vi "AcquireBurstModeData.vi"(7 "Watchdog":refnum<data-value>, 8 "error in (no error)":errorcluster, 11 "config in":T5 {"HighPassFilterState"."Filter State" format="%.2f"; "HighPassFilterState"."IIR Filter Cluster"."Forward Coefficients" format="%.2f"; "HighPassFilterState"."IIR Filter Cluster"."Reverse Coefficients" format="%.2f"; "FixedSizeX32"."InputConfig" items=["AC Coupled", "DC Coupled", "IEPE AC Coupled"]}) -> (0 "error out":errorcluster, 1 "burst mode dataflow messages":T1[](array[typedef]), 3 "config out":T5 {"HighPassFilterState"."Filter State" format="%.2f"; "HighPassFilterState"."IIR Filter Cluster"."Forward Coefficients" format="%.2f"; "HighPassFilterState"."IIR Filter Cluster"."Reverse Coefficients" format="%.2f"; "FixedSizeX32"."InputConfig" items=["AC Coupled", "DC Coupled", "IEPE AC Coupled"]})   [LabVIEW 2017, in "CmsAcquisition.lvlib"]
uses:
  <vilib>/addons/InsightCM/Devices/Shared/Cms/CmsAcquisition/CmsAcquisition.lvlib
  <vilib>/addons/InsightCM/Devices/Shared/Cms/CmsAcquisition/controls/Configuration.ctl
  <vilib>/addons/InsightCM/Devices/Shared/Cms/CmsAcquisition/controls/TachometerConfig.ctl
  <vilib>/addons/InsightCM/Devices/Shared/Cms/CmsAcquisition/controls/FixedSizeArrays.ctl
  <vilib>/LabVIEW Targets/FPGA/cRIO/shared/nicrio_ModuleControls/nicrio_cRIO-9232_ConfigModeRing.ctl
  <vilib>/addons/InsightCM/Devices/Shared/Cms/cRIOWfmAcq/subVIs/RIO Wfm Cust Ctrls/rwfm_SamplingInfo.ctl
  <vilib>/addons/InsightCM/Devices/Shared/Cms/CmsAcquisition/controls/Group.ctl
  <vilib>/addons/InsightCM/Devices/Shared/Cms/CmsAcquisition/controls/Channel.ctl
  <vilib>/addons/InsightCM/Utilities/Analysis/Vibration/controls/HighPassFilterState.ctl
  <vilib>/addons/InsightCM/Devices/Shared/Cms/CmsAcquisition/controls/BurstMode.ctl
  <vilib>/addons/InsightCM/Devices/Shared/Common/DataFlow/controls/Data.ctl
  <vilib>/addons/InsightCM/Utilities/DataAccessors/controls/wfmSGL_DVR.ctl
  <vilib>/addons/PointValueMap/controls/PointMap.ctl
  <vilib>/addons/InsightCM/Devices/Shared/Common/DataFlow/controls/Type.ctl
  <vilib>/NI/Software Watchdog/Watchdog/Watchdog.lvclass
  <vilib>/addons/InsightCM/Utilities/Analysis/Shared/controls/PulsePositions.ctl
  <vilib>/addons/InsightCM/Utilities/Analysis/Shared/AnalysisHelper.lvlib
  <vilib>/addons/PointValueMap/PointValueMap.lvlib
  <vilib>/addons/InsightCM/Devices/Shared/Common/DataFlow/DataFlow.lvlib
  <vilib>/addons/InsightCM/Devices/Shared/Cms/cRIOWfmAcq/cRIOWfmLib.lvlib
  <vilib>/addons/InsightCM/Utilities/Analysis/Vibration/VibrationAnalysisFunctions.lvlib
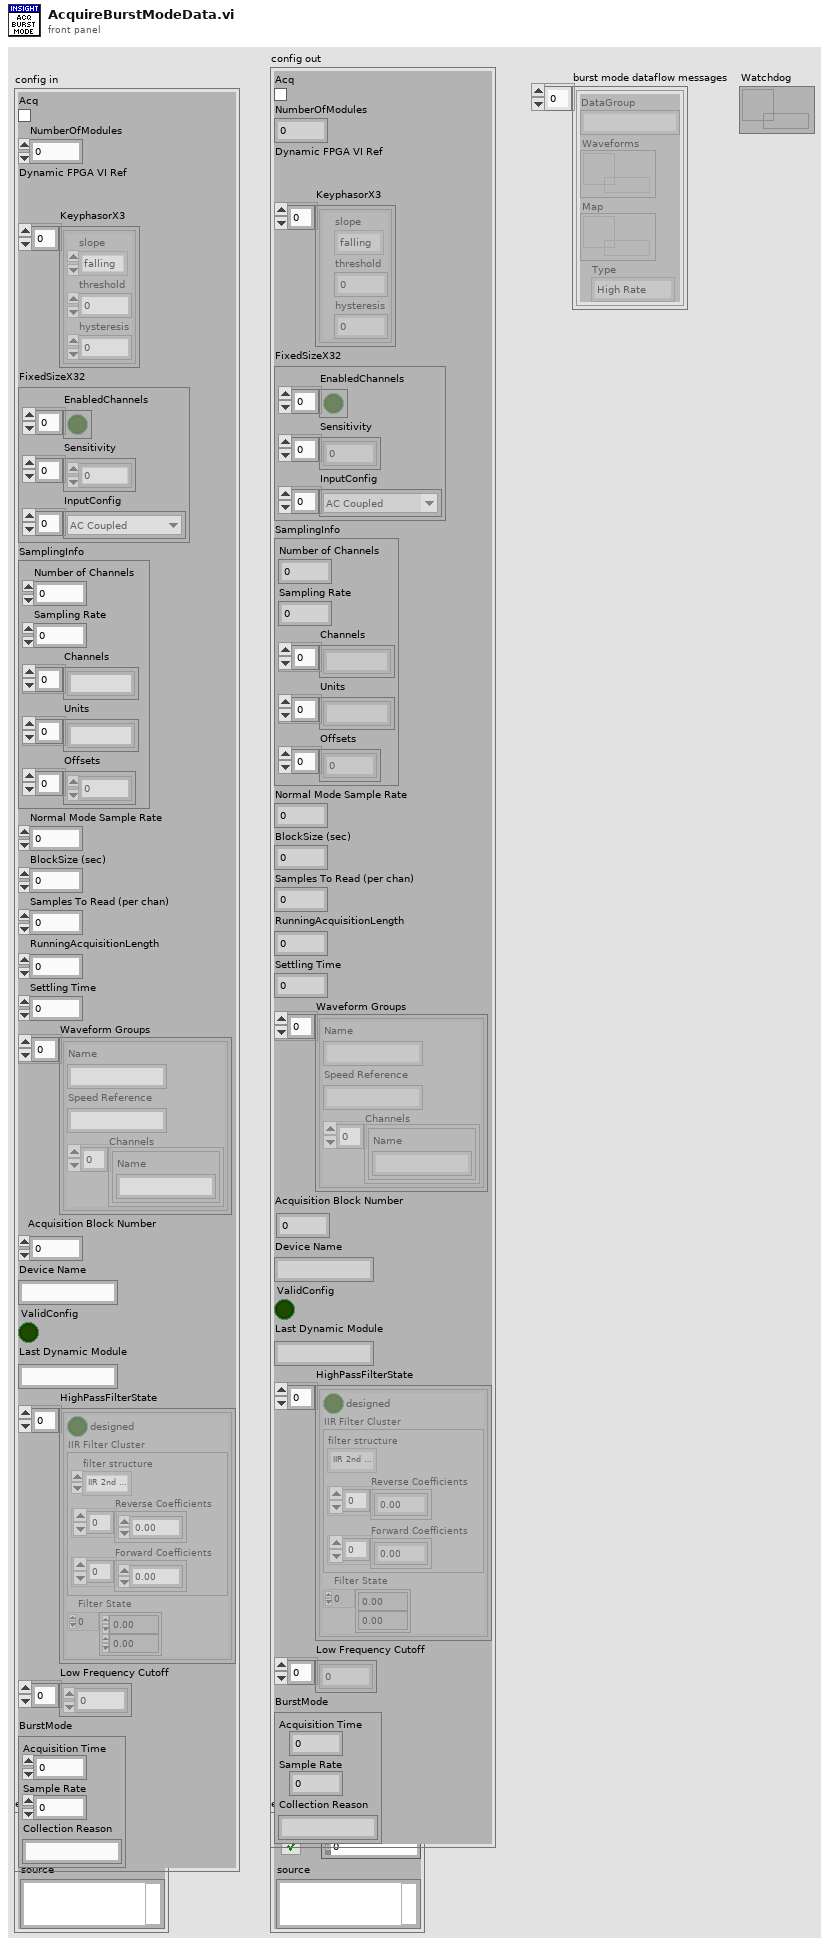
[diagram p1: front panel]
types:
  T1 = typedef "DataFlow.lvlib/Data.ctl" = cluster{"DataGroup":string, "Waveforms":T2, "Map":T3, "Type":T4}
  T2 = typedef "wfmSGL_DVR.ctl" = refnum<data-value>
  T3 = typedef "PointValueMap.lvlib/PointMap.ctl" = refnum<data-value>
  T4 = typedef "DataFlow.lvlib/Type.ctl" = enum16{"High Rate", "Low Rate", "Burst Mode"}
  T5 = typedef "CmsAcquisition.lvlib/Configuration.ctl" = cluster{"Acq":bool, "NumberOfModules":i16, "Dynamic FPGA VI Ref":refnum<k20>, "KeyphasorX3":T6[], "FixedSizeX32":T7, "SamplingInfo":T9, "Normal Mode Sample Rate":dbl, "BlockSize (sec)":dbl, "Samples To Read (per chan)":i32, "RunningAcquisitionLength":dbl, "Settling Time":dbl, "Waveform Groups":T10[], "Acquisition Block Number":i32, "Device Name":string, "ValidConfig":bool, "Last Dynamic Module":string, "HighPassFilterState":T12[], "Low Frequency Cutoff":dbl[], "BurstMode":T13}
  T6 = typedef "CmsAcquisition.lvlib/TachometerConfig.ctl" = cluster{"slope":enum16{"falling", "rising"}, "threshold":dbl, "hysteresis":dbl}
  T7 = typedef "CmsAcquisition.lvlib/FixedSizeArrays.ctl" = cluster{"EnabledChannels":bool[], "Sensitivity":dbl[], "InputConfig":T8[]}
  T8 = typedef "nicrio_cRIO-9232_ConfigModeRing.ctl" = u8
  T9 = typedef "cRIOWfmLib.lvlib/rwfm_SamplingInfo.ctl" = cluster{"Number of Channels":i32, "Sampling Rate":dbl, "Channels":string[], "Units":string[], "Offsets":sgl[]}
  T10 = typedef "CmsAcquisition.lvlib/Group.ctl" = cluster{"Name":string, "Speed Reference":string, "Channels":T11[]}
  T11 = typedef "CmsAcquisition.lvlib/Channel.ctl" = cluster{"Name":string}
  T12 = typedef "VibrationAnalysisFunctions.lvlib/HighPassFilterState.ctl" = cluster{"designed":bool, "IIR Filter Cluster":cluster{"filter structure":enum32{"IIR 2nd Order", "IIR 4th Order"}, "Reverse Coefficients":dbl[], "Forward Coefficients":dbl[]}, "Filter State":dbl[]}
  T13 = typedef "CmsAcquisition.lvlib/BurstMode.ctl" = cluster{"Acquisition Time":dbl, "Sample Rate":dbl, "Collection Reason":string}
  T14 = typedef "AnalysisHelper.lvlib/PulsePositions.ctl" = cluster{"Name":string, "Pulse Position Data":dbl[], "Pulses Per Rev":i32}
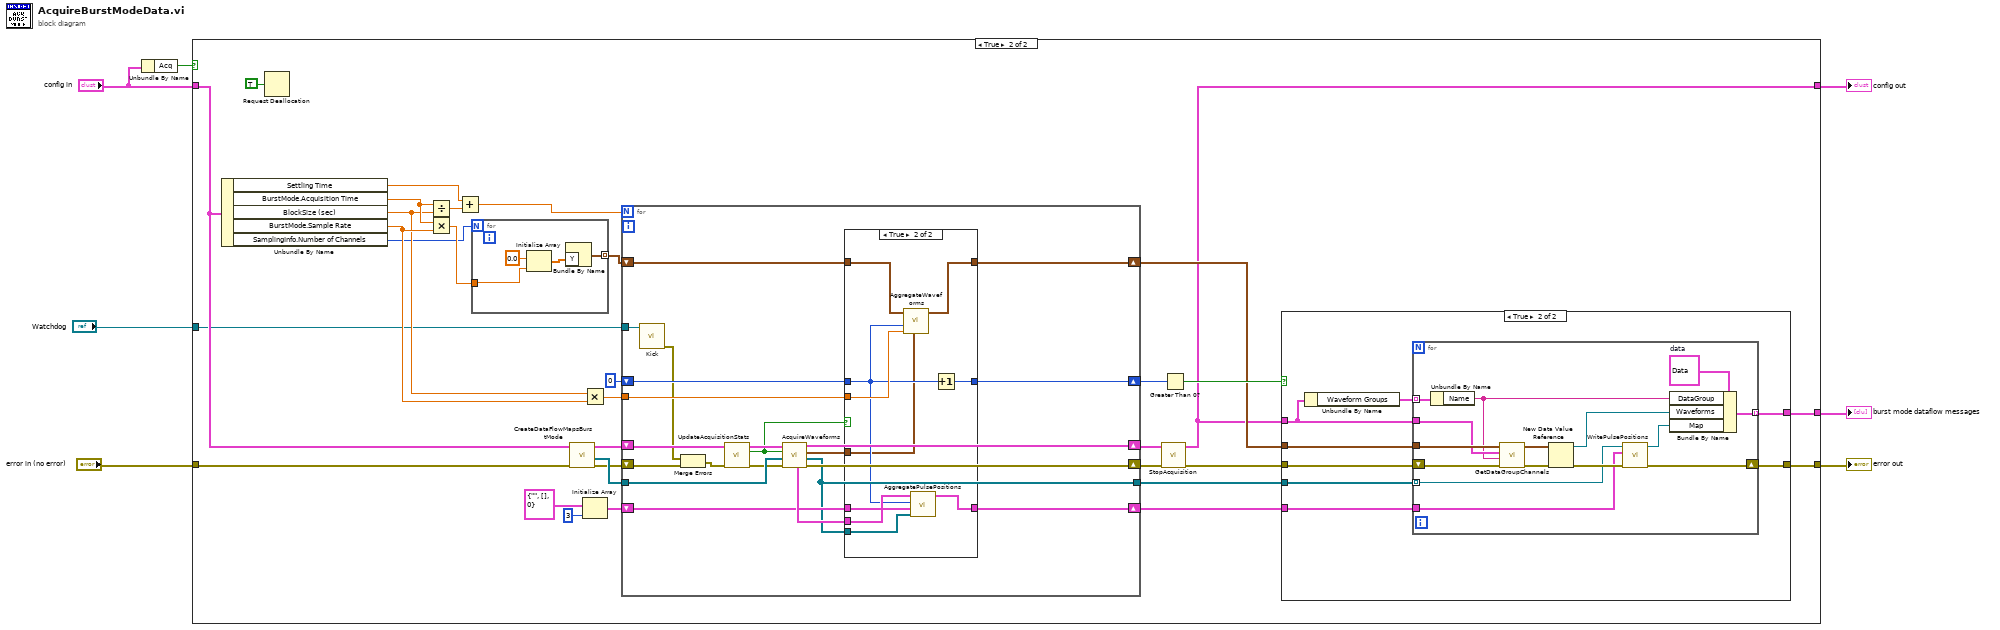
[diagram p0: block diagram]
diagram:
  n1 = Unbundle By Name("config in") -> ("Acq"=w5:bool)
  n2 = case shown="True" w5 {
    tunnel: "error in (no error)" -> [w9 w22]
    tunnel: "config in" -> [w8 w24]
    tunnel: [w8 w10] -> w4
    tunnel: [w9 w31] -> w3
    tunnel: [_ w29] -> w2
    tunnel: "Watchdog" -> [_ w18]
    frame False {
    }
    frame True {
      n3 = Unbundle By Name(w24) -> ("Settling Time"=w41:dbl, "BurstMode.Acquisition Time"=w39:dbl, "BlockSize (sec)"=w34:dbl, "BurstMode.Sample Rate"=w35:dbl, "SamplingInfo.Number of Channels"=w27:i32)
      n4 = Request Deallocation(TRUE ("flag")) -> ()
      n5 = Divide(x=w39, y=w34) -> (x/y=w40:dbl)
      n6 = Multiply(x=w39, y=w35) -> (x*y=w38:dbl)
      n7 = Add(x=w41, y=w40) -> (x+y=w28:dbl)
      n8 = for {
        N: w27 -> [_]
        tunnel: w38 -> [w44]
        tunnel: [w45] -> w37 mode=indexing
        n9 = Initialize Array(sgl 0.0 ("element"), w44) -> (w43:sgl[])
        n10 = Bundle By Name("Y"=w43) -> (w45:waveform(sgl))  [unwired: 1 in]
      }
      n11 = call <vilib>:"CreateDataFlowMapsBurstMode.vi"("error in (no error)"=w22, "923x Acquisition Config"=w24) -> ("error out"=w21:errorcluster, "maps"=w25:T3[], "923x Acquisition Config out"=w23:T5)  [unwired: 7 in]
      n12 = Multiply(x=w34, y=w35) -> (x*y=w33:dbl)
      n13 = Initialize Array(T14 {"Name"="", "Pulse Position Data"=[], "Pulses Per Rev"=0} ("Tachometer Pulses"), 3 ("dimension size")) -> (w32:T14[])
      n14 = for {
        N: w28 -> [_]
        shift-right: [w62] -> w15
        shift-left: 0 -> [w63]
        tunnel: w33 -> [w61]
        shift-right: [w48] -> w30
        shift-left: w32 -> [w60]
        shift-right: [w46] -> w12
        shift-left: w37 -> [w64]
        shift-right: [w59] -> w11
        shift-left: w23 -> [w58]
        shift-right: [w57] -> w20
        shift-left: w21 -> [w51]
        tunnel: [w53] -> w26
        tunnel: w25 -> [w56]
        tunnel: w18 -> [w52]
        n15 = call <vilib>:"Kick.vi"("Watchdog"=w52) -> ("error out"=w50:errorcluster)  [unwired: 9 in, 1 out]
        n16 = Merge Errors(w50, w51) -> (w49:errorcluster)
        n17 = call <vilib>:"UpdateAcquisitionStats.vi"("error in (no error)"=w49, "configuration"=w58) -> ("error out"=w54:errorcluster, "settling time requirement met?"=w47:bool, "configuration"=w55:T5)  [unwired: 7 in]
        n18 = call <vilib>:"AcquireWaveforms.vi"("error in (no error)"=w54, "Data Flow Maps"=w56, "settling time met"=w47, "923x Acquisition Config"=w55) -> ("error out"=w57:errorcluster, "Data Flow Maps out"=w53:T3[], "Waveforms"=w66:waveform(sgl)[], "923x Acquisition Config out"=w59:T5, "Pulse Positions Array"=w65:T14[])  [unwired: 3 in]
        n19 = case shown="True" w47 {
          tunnel: w66 -> [_ w70]
          tunnel: w65 -> [_ w72]
          tunnel: w64 -> [w68 w76]
          tunnel: w63 -> [w69 w73]
          tunnel: [w69 w78] -> w62
          tunnel: w61 -> [_ w75]
          tunnel: [w68 w79] -> w46
          tunnel: [w67 w77] -> w48
          tunnel: w60 -> [w67 w74]
          tunnel: w53 -> [_ w71]
          frame False {
          }
          frame True {
            n20 = call <vilib>:"AggregateWaveforms.vi"("new waveforms"=w70, "samples per block"=w75, "block count"=w73, "aggregate waveforms"=w76) -> ("aggregate waveforms out"=w79:waveform(sgl)[])  [unwired: 7 in]
            n21 = call <vilib>:"AggregatePulsePositions.vi"("data flow maps"=w71, "new pulse positions array"=w72, "block count"=w73, "pulse positions array aggregate"=w74) -> ("pulse positions array aggregate out"=w77:T14[])  [unwired: 7 in]
            n22 = Increment(x=w73) -> (x+1=w78:i32)
          }
        }
      }
      n23 = call <vilib>:"StopAcquisition.vi"("error in (no error)"=w20, "config"=w11) -> ("error out"=w19:errorcluster, "config out"=w10:T5)  [unwired: 8 in]
      n24 = Greater Than 0?(x=w15) -> (x > 0?=w13:bool)
      n25 = case shown="True" w13 {
        tunnel: w26 -> [_ w88]
        tunnel: w19 -> [w80 w87]
        tunnel: [w80 w86] -> w31
        tunnel: [_ w85] -> w29
        tunnel: w30 -> [_ w84]
        tunnel: w10 -> [_ w83]
        tunnel: w12 -> [_ w81]
        frame False {
        }
        frame True {
          n26 = Unbundle By Name(w83) -> ("Waveform Groups"=w82:T10[])
          n27 = for {
            tunnel: w82 -> [w91] mode=indexing
            tunnel: w81 -> [w92]
            tunnel: w84 -> [w99]
            tunnel: w88 -> [w96] mode=indexing
            tunnel: [w103] -> w85 mode=indexing
            shift-right: [w97] -> w86
            shift-left: w87 -> [w94]
            tunnel: w83 -> [w90]
            w102 = T1 {"DataGroup"="", "Waveforms"=refnum, "Map"=refnum, "Type"=enum."High Rate"}  # data
            n28 = Unbundle By Name(w91) -> ("Name"=w89:string)
            n29 = call <vilib>:"GetDataGroupChannels.vi"("error in (no error)"=w94, "group"=w89, "923x acquisition config"=w90, "all waveforms"=w92) -> ("error out"=w95:errorcluster, "this groups channels"=w93:waveform(sgl)[])  [unwired: 6 in]
            n30 = New Data Value Reference(data value=w93, error in=w95) -> (data value reference=w101:refnum<data-value>, error out=w100:errorcluster)
            n31 = call <vilib>:"WritePulsePositions.vi"("error in (no error)"=w100, "pulse positions array"=w99, "map in"=w96) -> ("error out"=w97:errorcluster, "map out"=w98:T3)  [unwired: 7 in]
            n32 = Bundle By Name(cluster=w102, "DataGroup"=w89, "Waveforms"=w101, "Map"=w98) -> (w103:T1)
          }
        }
      }
    }
  }
  "error out" <- w3
  "config out" <- w4
  "burst mode dataflow messages" <- w2
